vi "RSZVB Set Calculation of Bandfilter Center Frequency.vi"(7 "Center Frequency Calculation (Geometric)":i32(ring) items=["Geometric", "Arithmetic"], 8 "error in (no error)":errorcluster {"code" format="%.0x"}, 9 "Marker (1)":i32=1, 10 "Channel (1)":i32=1, 11 "VISA session":refnum<visa-resource-name>) -> (0 "error out":errorcluster {"code" format="%.0x"}, 3 "dup VISA session":refnum<visa-resource-name>)   [LabVIEW 2011]
doc: "This VI specifies how the center frequency of a bandfilter search is calculated.\n\nRemote-control command(s):\nCALCulate<Chn>:MARKer<Mk>:FUNCtion:BWIDth:GMCenter <Boolean>"
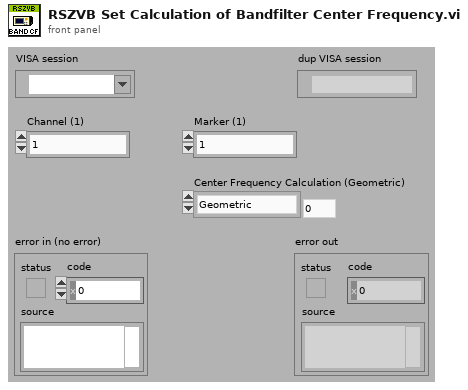
[diagram p1: front panel]
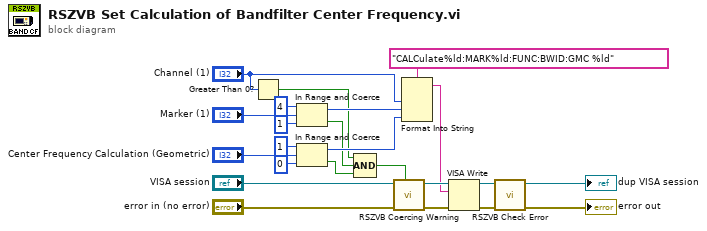
[diagram p0: block diagram]
diagram:
  n1 = Greater Than 0?(x="Channel (1)") -> (x > 0?=w7:bool)
  n2 = In Range and Coerce(upper limit=4, x="Marker (1)", lower limit=1) -> (coerced(x)=w10:i32, In Range?=w6:bool)
  n3 = In Range and Coerce(upper limit=1, x="Center Frequency Calculation (Geometric)", lower limit=0) -> (coerced(x)=w9:i32, In Range?=w5:bool)
  n4 = Compound Arithmetic op=AND(w7, w6, w5) -> (w4:bool)
  n5 = call "RSZVB Coercing Warning.vi"("In Range?"=w4, "error in (no error)"="error in (no error)", "VISA session"="VISA session") -> ("error out"=w21:errorcluster, "dup VISA session"=w22:refnum<visa-resource-name>)  [unwired: 7 in]
  n6 = Format Into String(format string="CALCulate%ld:MARK%ld:FUNC:BWID:GMC %ld", "Channel (1)", w10, w9) -> (resulting string=w20:string)  [unwired: 2 in, 1 out]
  n7 = VISA Write(VISA resource name=w22, write buffer=w20, error in (no error)=w21) -> (VISA resource name out=w12:refnum<visa-resource-name>, error out=w11:errorcluster)  [unwired: 1 out]
  n8 = call "RSZVB Check Error.vi"("error in (no error)"=w11, "VISA session"=w12) -> ("error out"=→"error out":errorcluster, "dup VISA session"=→"dup VISA session":refnum<visa-resource-name>)  [unwired: 8 in]
